vi "M9003Open.vi"() -> (0 "HANDLE":i32)   [LabVIEW 2009]
uses:
  M9003api.dll
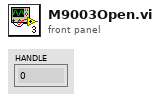
[diagram p1: front panel]
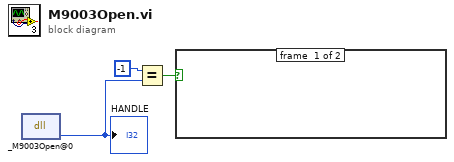
[diagram p0: block diagram]
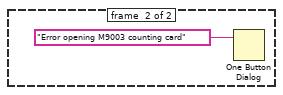
[diagram p2: hidden frame]
diagram:
  n1 = dll-call lib="H:/Mover_2009/Sub_Vis/M9003Commands/M9003api.dll" fn="_M9003Open@0" label="M9003Open"() -> ("Handle"=w2:i32)  [unwired: 3 in, 2 out]
  "HANDLE" <- w2
  n2 = Equal?(x=-1, y=w2) -> (x = y?=w3:bool)
  n3 = case shown="True" w3 {
    frame #0 {
    }
    frame #1 {
      n4 = One Button Dialog(message="Error opening M9003 counting card") -> ()  [unwired: 1 in, 1 out]
    }
  }
